vi "LoadCore.vi"(8 "error in (no error)":errorcluster, 10 "ErrorDetails":string[][](array[string]), 11 "LabErrorUX in":refnum<class "LabErrorUX.lvclass">) -> (0 "error out":errorcluster, 3 "LabErrorUX out":refnum<class "LabErrorUX.lvclass">)   [LabVIEW 2019, in "LabErrorUX.lvclass"]
uses:
  LabErrorUX.lvclass
  LabErrorUX.lvclass/LabErrorUX.ctl
  <vilib>/SLL Toolkit/SLL Table/SLL Table.lvclass
  Typedefs/ErrorUX.ctl
  <vilib>/SLL Toolkit/SLL Table/_SubVIs/Get Row Data.vi
  <vilib>/SLL Toolkit/SLL Table/_SubVIs/Get Cell Data.vi
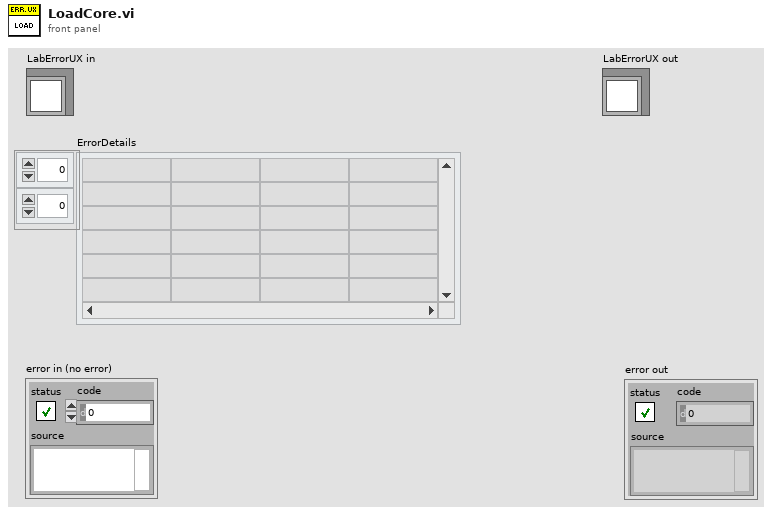
[diagram p1: front panel]
types:
  T1 = typedef "LabErrorUX.lvclass/ErrorUX.ctl" = cluster{"Code":string, "Format":string, "Title":string, "Reason":string, "Next Steps":string, "Web Help":string, "Local Help":string, "Info Map":map{string, string}, "Format Tags":map{string, string}}
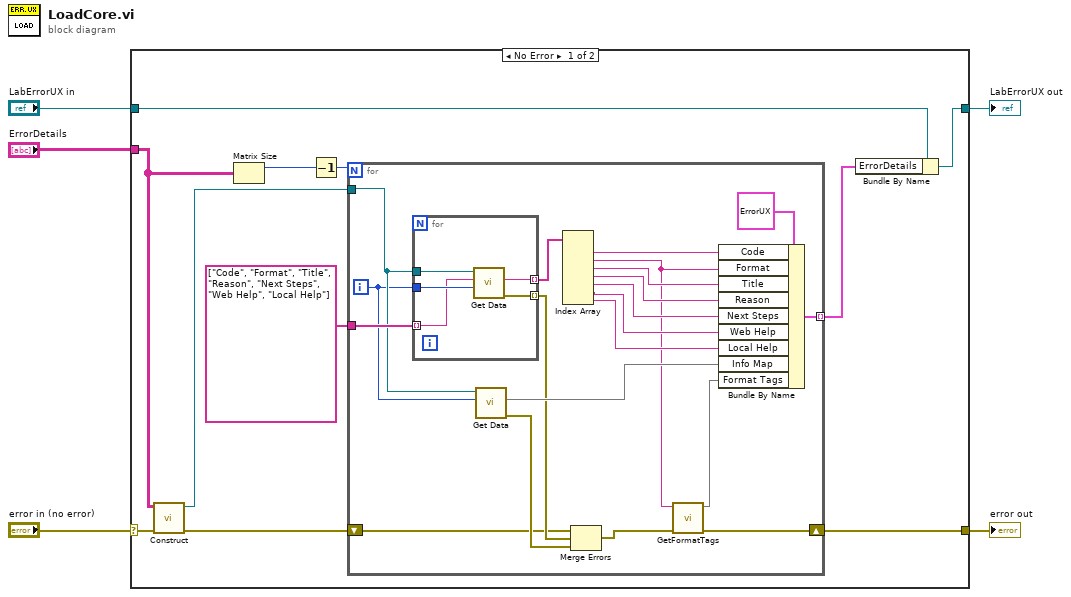
[diagram p0: block diagram]
diagram:
  n1 = case shown="No Error" "error in (no error)" {
    selector: "error in (no error)" -> [w8 w43]
    tunnel: [w6 w43] -> w4
    tunnel: [w15 w42] -> w2
    tunnel: "LabErrorUX in" -> [w16 w42]
    tunnel: "ErrorDetails" -> [w13 _]
    frame No Error {
      n2 = call <vilib>:"Construct.vi"("error in (no error)"=w8, "2D String with Headers"=w13) -> ("error out"=w7:errorcluster, "Table"=w14:refnum<class "SLL Table.lvclass">)  [unwired: 8 in]
      n3 = Matrix Size(0:w13) -> (1:w12:i32)  [unwired: 1 out]
      n4 = Decrement(x=w12) -> (x-1=w11:i32)
      n5 = for {
        N: w11 -> [_]
        tunnel: w14 -> [w29]
        tunnel: string[] ["Code", "Format", "Title", "Reason", "Next Steps", "Web Help", "Local Help"] -> [w35]
        tunnel: [w31] -> w9 mode=indexing
        shift-right: [w17] -> w6
        shift-left: w7 -> [w18]
        i -> [w28]
        n6 = for {
          tunnel: w29 -> [w38]
          tunnel: w28 -> [w41]
          tunnel: w35 -> [w40] mode=indexing
          tunnel: [w39] -> w34 mode=indexing
          tunnel: [w37] -> w22 mode=indexing
          n7 = call-poly <vilib>:"Get Data.vi"("Row Index"=w41, "Header"=w40, "SLL Table in"=w38) -> ("error out"=w37:errorcluster, "Cell Data"=w39:string)  [unwired: 5 in, 2 out]
        }
        n8 = call-poly <vilib>:"Get Data.vi"("Row Index"=w28, "SLL Table in"=w29) -> ("error out"=w21:errorcluster, "Row Map"=w27:map{string, string})  [unwired: 7 in, 1 out]
        n9 = Index Array(array=w34) -> (element #1=w30:string, element #2=w23:string, element #3=w33:string, element #4=w32:string, element #5=w26:string, element #6=w25:string, element #7=w24:string)  [unwired: 7 in]
        n10 = Merge Errors(w18, w22, w21) -> (w20:errorcluster)
        n11 = call "GetFormatTags.vi"("error in (no error)"=w20, "Format String"=w23) -> ("error out"=w17:errorcluster, "Format Tags"=w19:map{string, string})  [unwired: 8 in]
        n12 = Bundle By Name(cluster=T1 {"Code"="", "Format"="", "Title"="", "Reason"="", "Next Steps"="", "Web Help"="", "Local Help"="", "Info Map"={}, "Format Tags"={}} ("ErrorUX"), "Code"=w30, "Format"=w23, "Title"=w33, "Reason"=w32, "Next Steps"=w26, "Web Help"=w25, "Local Help"=w24, "Info Map"=w27, "Format Tags"=w19) -> (w31:T1)
      }
      n13 = Bundle By Name(cluster=w16, "ErrorDetails"=w9) -> (w15:refnum<class "LabErrorUX.lvclass">)
    }
    frame Error {
    }
  }
  "error out" <- w4
  "LabErrorUX out" <- w2
